vi "Dynamic call-Funct img viewer (rectangles).vi"(8 "error in (no error)":errorcluster, 11 "Experiment Path":path) -> (0 "error out":errorcluster)   [LabVIEW 2020]
uses:
  Visualisation/Timelapse Viewer/Globals/gl_Time series viewer globals.vi
  Global Variables/General Globals.vi
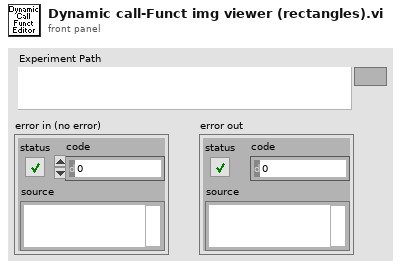
[diagram p1: front panel]
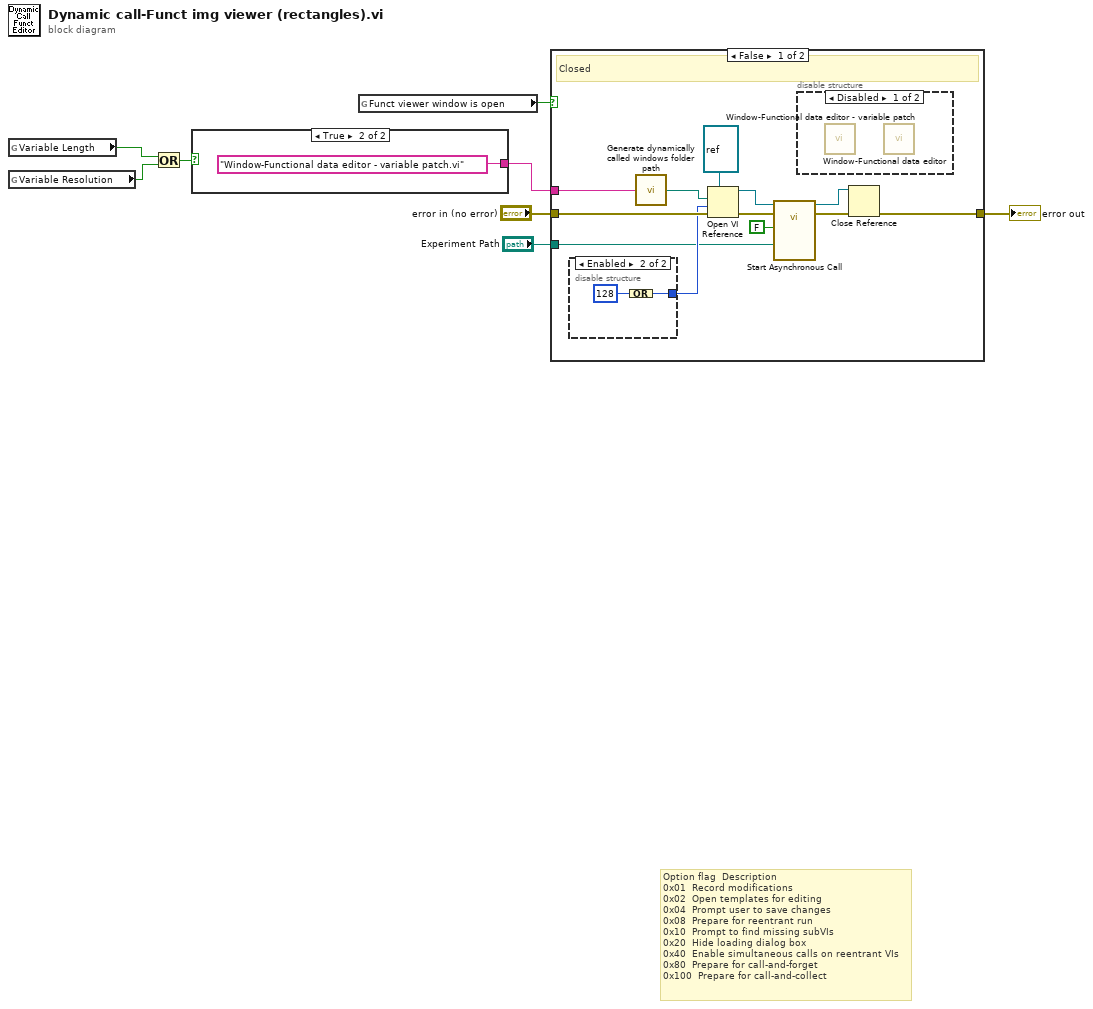
[diagram p0: block diagram]
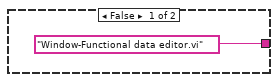
[diagram p2: hidden frame]
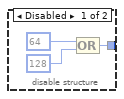
[diagram p3: hidden frame]
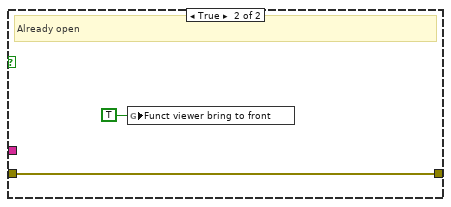
[diagram p5: hidden frame]
diagram:
  # "Option flag \tDescription\n0x01 \tRecord modifications\n0x02 \tOpen templates for editing\n0x04 \tPrompt user to save changes\n0x08 \tPrepare for reentrant run\n0x10 \tPrompt to find missing subVIs\n0x20 \tHide loading dialog box\n0x40 \tEnable simultaneous calls on reentrant VIs\n0x80 \tPrepare for call-and-forget\n0x100 \tPrepare for call-and-collect"
  n1 = global read "General Globals.vi" "Variable Length"() -> (w3:bool)
  n2 = global read "General Globals.vi" "Variable Resolution"() -> (w2:bool)
  n3 = Or(x=w3, y=w2) -> (x .or. y?=w1:bool)
  n4 = case shown="True" w1 {
    tunnel: ["Window-Functional data editor.vi" ("Error Source") "Window-Functional data editor - variable patch.vi" ("Error Source")] -> w4
    frame False {
    }
    frame True {
    }
  }
  n5 = global read "gl_Time series viewer globals.vi" "Funct viewer window is open"() -> (w6:bool)
  n6 = case shown="False" w6 {
    tunnel: "error in (no error)" -> [w22 w28]
    tunnel: [w21 w28] -> w7
    tunnel: w4 -> [w19 _]
    tunnel: "Experiment Path" -> [w11 _]
    frame False {
      # "Closed"
      n7 = disable-structure shown="Enabled" {
        disable-tunnel: [w25 w27] -> w16
        frame Disabled {
          n8 = Compound Arithmetic op=OR(64, 128) -> (w25:i32)
        }
        frame Enabled {
          n9 = Compound Arithmetic op=OR(128) -> (w27:i32)
        }
      }
      n10 = call "Generate dynamically called windows folder path.vi"("name of dynamically called VI"=w19) -> ("Dynamically called VI path"=w20:path)
      n11 = Open VI Reference(type specifier VI Refnum (for type only)=refnum<vi> refnum, vi path=w20, options=w16, error in (no error)=w22) -> (vi reference=w17:refnum<vi>, error out=w18:errorcluster)  [unwired: 2 in]
      n12 = call-by-ref "Start Asynchronous Call"(reference=w17, error in=w18, "Experiment Path"=w11, "Standalone viewer?"=FALSE) -> (reference out=w13:refnum<vi>, error out=w14:errorcluster)  [unwired: 10 in]
      n13 = disable-structure shown="Disabled" {
        frame Disabled {
          n14 = call "Window-Functional data editor.vi"() -> ()  [unwired: 12 in]
          n15 = call "Window-Functional data editor - variable patch.vi"() -> ()  [unwired: 12 in]
        }
        frame Enabled {
        }
      }
      n16 = Close Reference(reference=w13, error in (no error)=w14) -> (error out=w21:errorcluster)
    }
    frame True {
      # "Already open"
      n17 = global write "gl_Time series viewer globals.vi" "Funct viewer bring to front"(TRUE ("Bring Timelapse Editor to front")) -> ()
    }
  }
  "error out" <- w7
